vi "SVL Set dB Reference (N Ch - N Ref).vi"(8 "error in (no error)":errorcluster, 10 "dB references [EU]":dbl[](array[numeric]) format="%^.1e", 11 "scaled signals in [EU]":waveform(dbl)[](array[waveform])=[{"t0"=timestamp(0 s since 1904-01-01), "dt"=0.0, "Y"=[]}]) -> (0 "error out":errorcluster, 3 "scaled signals out [EU]":waveform(dbl)[](array[waveform]))   [LabVIEW 2017]
doc: "Sets the specified <B>dB reference [EU]</B> as an attribute in the <B>scaled signal out [EU]</B> waveform. <B>dB reference [EU]</B> is used for all downstream conversions to dB. Wire data to the <B>scaled signal in [EU]</B> input to determine the polymorphic instance to use or manually select the instance."
uses:
  <vilib>/addons/_NISVFA/_Shared subVIs/Common/SVL Set dB Reference (variant).vi
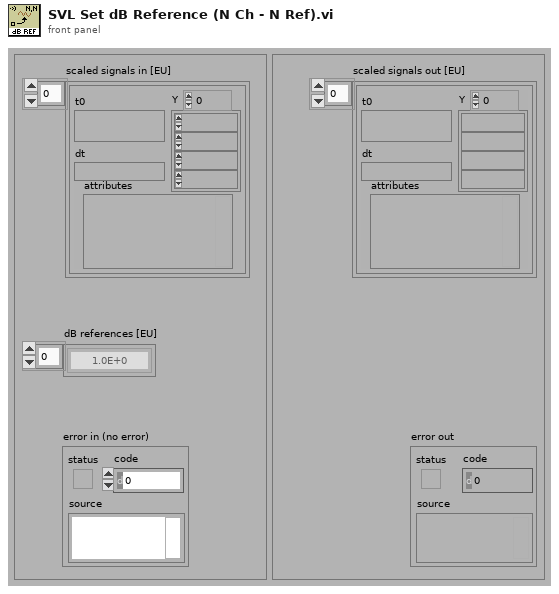
[diagram p1: front panel]
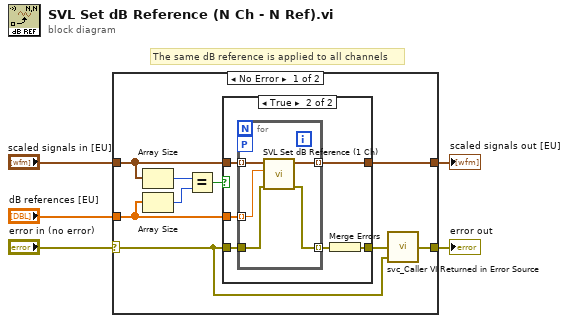
[diagram p0: block diagram]
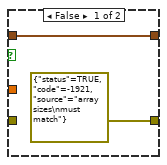
[diagram p2: hidden frame]
diagram:
  # "The same dB reference is applied to all channels"
  n1 = case shown="No Error" "error in (no error)" {
    selector: "error in (no error)" -> [w11 w29]
    tunnel: "scaled signals in [EU]" -> [w8 w28]
    tunnel: [w14 w29] -> w4
    tunnel: [w13 w28] -> w3
    tunnel: "dB references [EU]" -> [w7 _]
    frame No Error {
      n2 = Array Size(array=w8) -> (size(s)=w10:i32)
      n3 = Array Size(array=w7) -> (size(s)=w9:i32)
      n4 = Equal?(x=w10, y=w9) -> (x = y?=w6:bool)
      n5 = case shown="True" w6 {
        tunnel: [w16 w22] -> w13
        tunnel: [errorcluster {"status"=TRUE, "code"=-1921, "source"="array sizes\nmust match"} ("error IO") w17] -> w12
        tunnel: w11 -> [_ w20]
        tunnel: w8 -> [w16 w19]
        tunnel: w7 -> [_ w18]
        frame False {
        }
        frame True {
          n6 = for {
            tunnel: w19 -> [w27] mode=indexing
            tunnel: [w26] -> w22 mode=indexing
            tunnel: w18 -> [w25] mode=indexing
            tunnel: w20 -> [w23]
            tunnel: [w24] -> w21 mode=indexing
            workers-P: _ -> [_]
            n7 = call <vilib>:"SVL Set dB Reference (1 Ch).vi"("error in (no error)"=w23, "dB reference [EU]"=w25, "scaled signal in [EU]"=w27) -> ("error out"=w24:errorcluster, "scaled signal out [EU]"=w26:waveform(dbl))  [unwired: 7 in]
          }
          n8 = Merge Errors(w21) -> (w17:errorcluster)
        }
      }
      n9 = call <vilib>:"svc_Caller VI Returned in Error Source.vi"("warning input to caller"=w11, "error in (no error)"=w12) -> ("error out"=w14:errorcluster)  [unwired: 3 in]
    }
    frame Error {
    }
  }
  "scaled signals out [EU]" <- w3
  "error out" <- w4
